vi "模态分析使用版.vi"() -> ()   [LabVIEW 2014]
uses:
  <vilib>/Analysis/4window.llb/windowTd.ctl
  <vilib>/Analysis/3filter.llb/Filter Structure Type.ctl
  <vilib>/measure/macond.llb/IIR Filter for 1 Chan.vi
  <vilib>/Waveform/WDTOps.llb/WDT Number of Waveform Samples DBL.vi
  <vilib>/Waveform/WDTOps.llb/WDT Append Waveforms DBL.vi
  <vilib>/Waveform/WDTOps.llb/WDT Get Waveform Subset DBL.vi
  <vilib>/measure/maspectr.llb/Frequency Response Function (Mag-Phase) 1-1.vi
  <vilib>/measure/NI_MAPro.lvlib
  <vilib>/Analysis/NI_AALPro.lvlib
  <vilib>/Analysis/NI_AALBase.lvlib
panel:
  out "数组 4":dbl[](array[numeric])
  out "数组 3":dbl[](array[numeric])
  out "FRF magnifitude 10":dbl[](graph) caption="FRF magnifitude"
  out "FRF magnifitude 8":cluster{"f0":dbl, "df":dbl, "magnitude":dbl[]}(graph) caption="FRF magnifitude"
  out "FRF magnifitude 7":cluster{"f0":dbl, "df":dbl, "magnitude":dbl[]}(graph) caption="FRF magnifitude"
  in  "filter structure option":T1=10 caption="滤波器结构选项" items=["IIR二阶"=0, "IIR四阶"=1, "自动选择"=10]
  in  "IIR filter specifications":T2={"Topology"=enum."Butterworth", "Type"=enum."Lowpass", "Order"=5, "Lower Fc"=1000.0, "Upper Fc"=200.0, "PB Ripple"=1.0, "SB Attenuation"=60.0} caption="IIR滤波器规范" {"PB Ripple" format="%0.2f"; "SB Attenuation" format="%0.2f"; "Lower Fc" format="%0.2p"; "Upper Fc" format="%0.2p"}
  out "FRF magnifitude 6":waveform(dbl)(graph) caption="FRF magnifitude"
  in  "Real":dbl
  out "FRF magnifitude 5":dbl[](graph) caption="FRF magnifitude"
  out "FRF magnifitude 3":cluster{"f0":dbl, "df":dbl, "magnitude":dbl[]}(graph) caption="FRF magnifitude"
  out "FRF magnifitude 2":cluster{"f0":dbl, "df":dbl, "magnitude":dbl[]}(graph) caption="FRF magnifitude"
  out "相关函数 2":cluster{"f0":dbl, "df":dbl, "magnitude":dbl[]}(graph)
  out "FRF Phase 2":cluster{"f0":dbl, "df":dbl, "magnitude":dbl[]}(graph)
  in  "FRF Mode 2":enum16{"H1", "H2", "H3"}(ring) caption="FRF模式"
  in  "averaging parameters 2":T3={"averaging mode"=enum."No averaging", "weighting mode"=enum."Exponential", "number of averages"=10} caption="平均参数" {"number of averages" min=1}
  out "error out 2":errorcluster caption="错误输出"
  in  "error in (no error)":errorcluster caption="错误输入（无错误）"
  in  "view 2":T4 caption="查看"
  in  "window 2":T5=1 caption="窗" items=["矩形"=0, "Hanning"=1, "Hamming"=2, "Blackman-Harris"=3, "Exact Blackman"=4, "Blackman"=5, "Flat Top"=6, "4阶Blackman-Harris "=7, "7阶Blackman-Harris"=8, "Low Sidelobe"=9, "Blackman Nuttall"=11, "三角"=30, "Bartlett-Hanning"=31, "Bohman"=32, "Parzen"=33, "Welch"=34, "Kaiser"=60, "Dolph-Chebyshev"=61, "高斯"=62]
  out "最大值":dbl
  out "数组 2":dbl[](array[numeric])
  out "数组":dbl[](array[numeric])
  out "error out":errorcluster
  in  "数值":i32
  out "FRF magnifitude":cluster{"f0":dbl, "df":dbl, "magnitude":dbl[]}(graph)
  out "相关函数":cluster{"f0":dbl, "df":dbl, "magnitude":dbl[]}(graph)
  out "FRF Phase":cluster{"f0":dbl, "df":dbl, "magnitude":dbl[]}(graph)
  out "响应信号":waveform(dbl)(graph)
  out "激振信号":waveform(dbl)(graph)
  in  "averaging parameters":T3={"averaging mode"=enum."No averaging", "weighting mode"=enum."Exponential", "number of averages"=10} caption="平均参数" {"number of averages" min=1}
  in  "window":T5=1 caption="窗" items=["矩形"=0, "Hanning"=1, "Hamming"=2, "Blackman-Harris"=3, "Exact Blackman"=4, "Blackman"=5, "Flat Top"=6, "4阶Blackman-Harris "=7, "7阶Blackman-Harris"=8, "Low Sidelobe"=9, "Blackman Nuttall"=11, "三角"=30, "Bartlett-Hanning"=31, "Bohman"=32, "Parzen"=33, "Welch"=34, "Kaiser"=60, "Dolph-Chebyshev"=61, "高斯"=62]
  in  "view":T4 caption="查看"
  in  "FRF Mode":enum16{"H1", "H2", "H3"}(ring) caption="FRF模式"
  in  "删除上一次波形":bool
  in  "激振计数":i32=-1 caption="预触发长度"
  in  "阈值":dbl=-1.0
  in  "预触发长度":i32=-1
  in  "激振通道":i32=-1
  in  "激振传感器灵敏度":dbl=-1.0
  in  "采集次数":i32=-1 caption="预触发长度"
  in  "停止按钮":bool
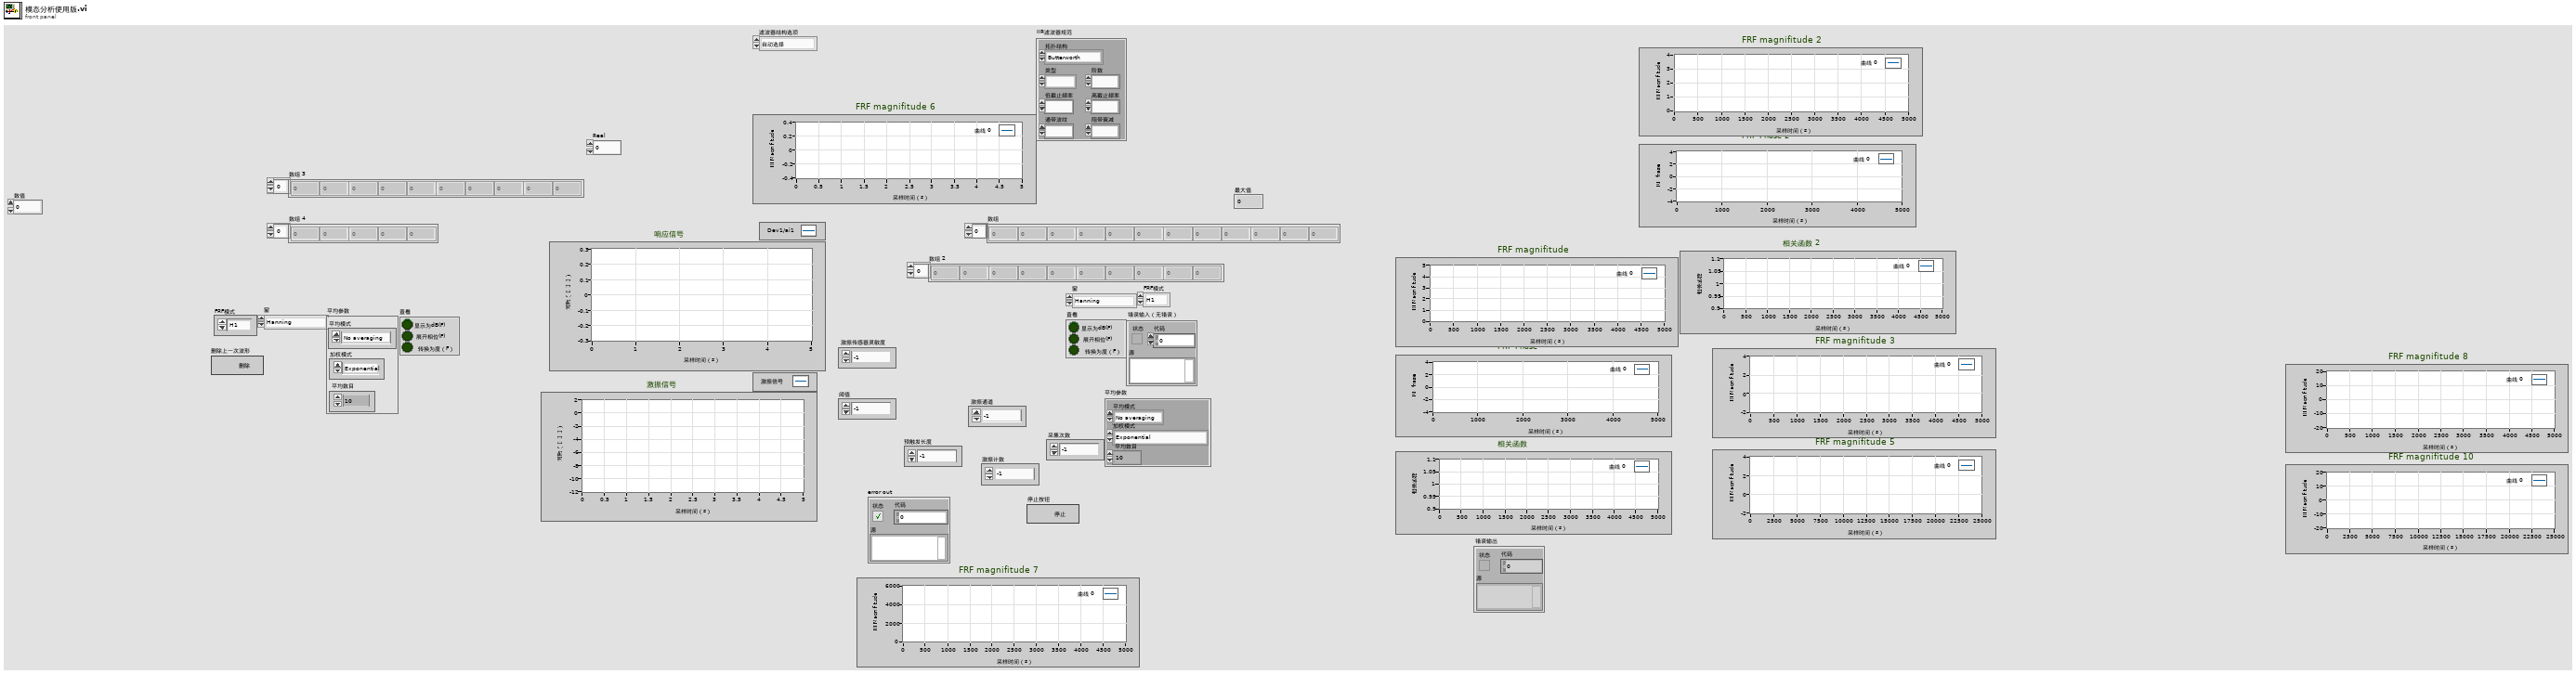
[diagram p1: front panel]
types:
  T1 = typedef "NI_AALBase.lvlib/Filter Structure Type.ctl" = u16
  T2 = cluster{"Topology":enum16{"Off", "Butterworth", "Chebyshev", "Inverse Chebyshev", "Elliptic", "Bessel"}, "Type":enum16{"Lowpass", "Highpass", "Bandpass", "Bandstop"}, "Order":i32, "Lower Fc":dbl, "Upper Fc":dbl, "PB Ripple":dbl, "SB Attenuation":dbl}
  T3 = cluster{"averaging mode":enum16{"No averaging", "Vector averaging", "RMS averaging", "Peak hold"}, "weighting mode":enum16{"Linear", "Exponential"}, "number of averages":u32}
  T4 = cluster{"dB On (F)":bool, "unwrap phase (F)":bool, "convert to degree (F)":bool}
  T5 = typedef "NI_AALPro.lvlib/windowTd.ctl" = u32
  T6 = cluster{"magnitude":cluster{"f0":dbl, "df":dbl, "magnitude":dbl[]}, "phase":cluster{"f0":dbl, "df":dbl, "phase":dbl[]}, "coherence":cluster{"f0":dbl, "df":dbl, "coherence":dbl[]}}
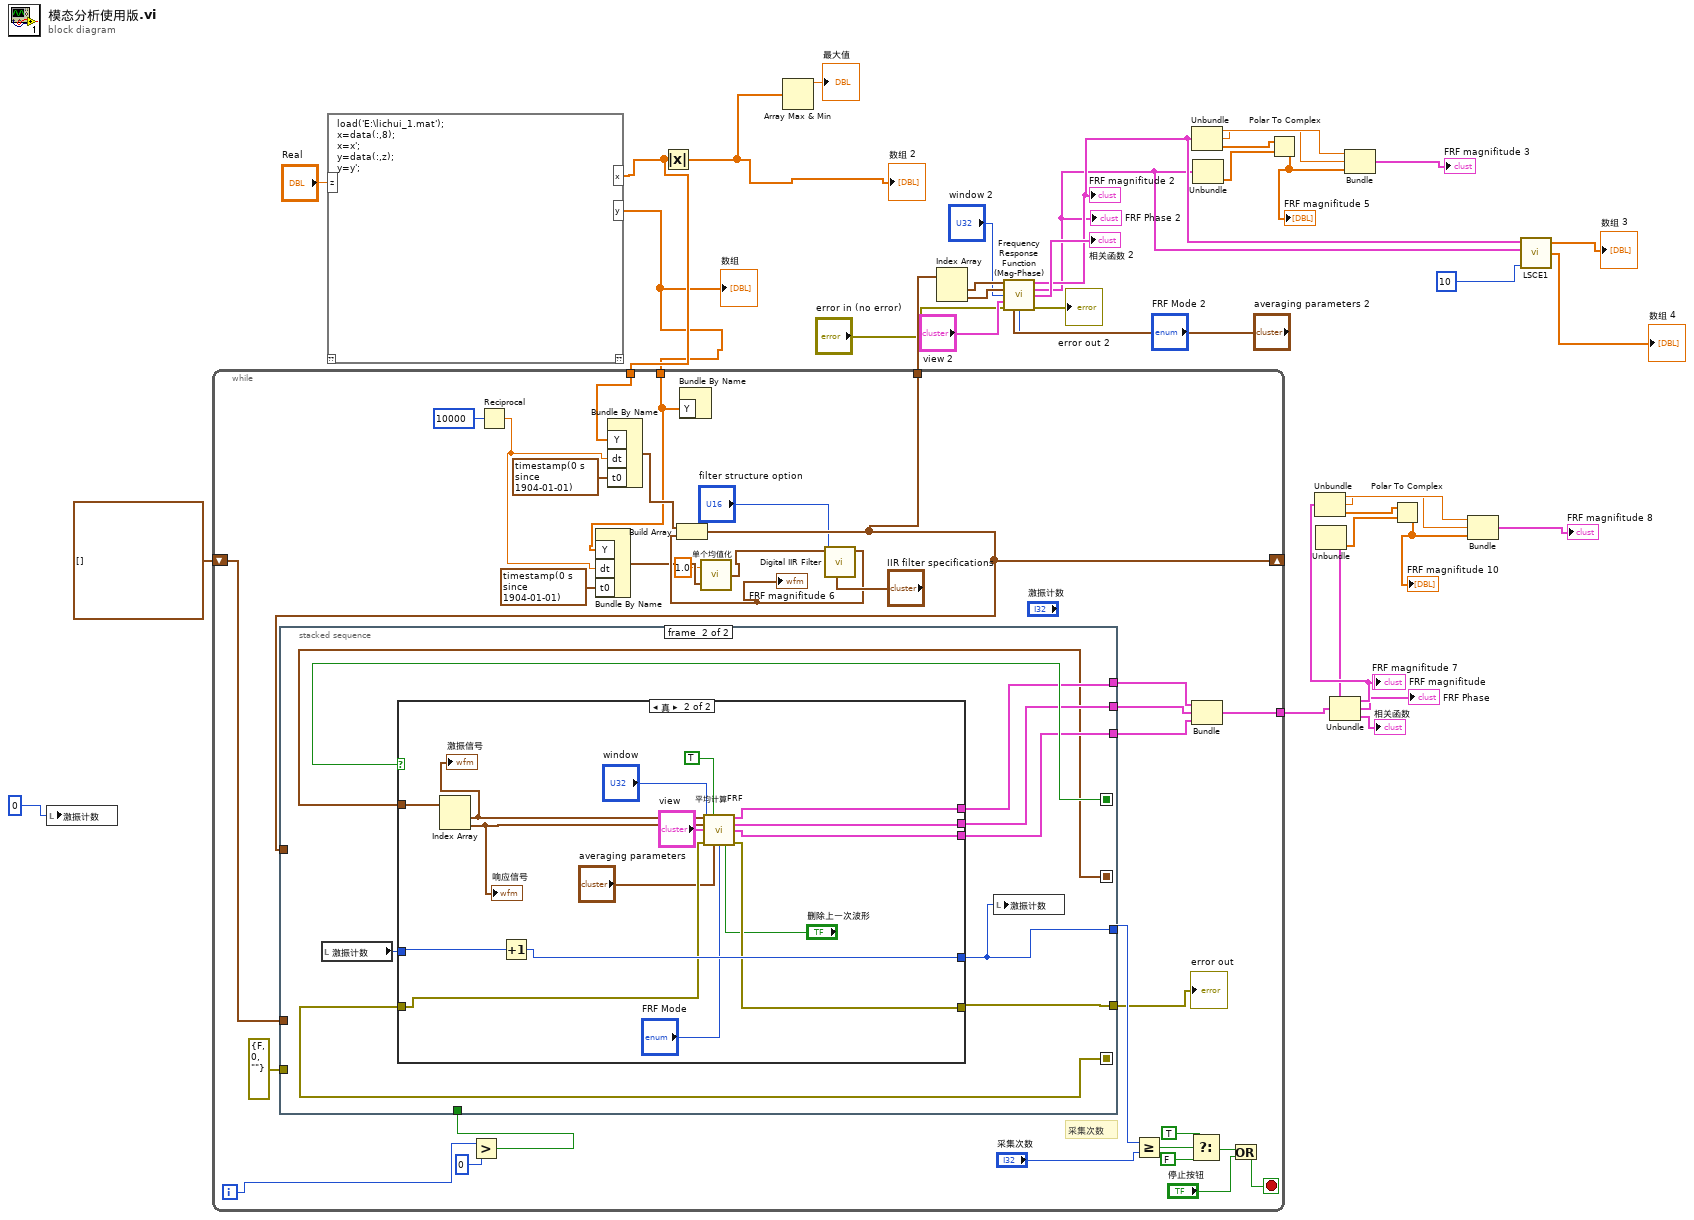
[diagram p0: block diagram]
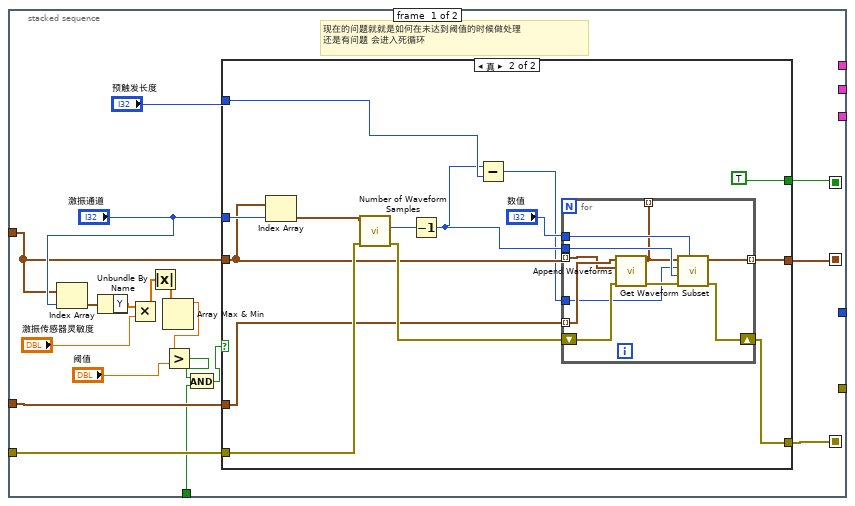
[diagram p2: hidden frame]
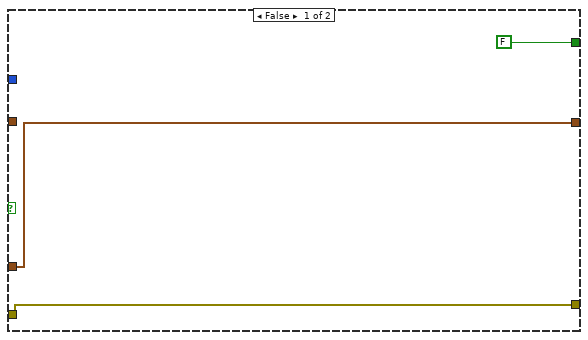
[diagram p3: hidden frame]
diagram:
  n1 = local write "激振计数"(0) -> ()
  n2 = script code="load('E:\\lichui_1.mat');\nx=data(:,8);\nx=x';\ny=data(:,z);\ny=y';"("z"="Real") -> ("x"=w15:dbl[], "y"=w14:dbl[])  [unwired: 1 in, 1 out]
  "数组" <- w14
  n3 = while {
    shift-right: [w47] -> _
    shift-left: waveform(dbl)[] [] ("data") -> [w70]
    tunnel: [w61] -> w35
    tunnel: w15 -> [w48]
    tunnel: w14 -> [w45]
    tunnel: [w47] -> w33
    i -> [w56]
    stop <- w59 stop-if-true
    # "采集次数"
    n4 = Greater?(x=w56, y=0) -> (0:w55:bool)
    n5 = Reciprocal(x=10000) -> (1/x=w49:dbl)
    n6 = Bundle By Name("Y"=w45, "dt"=w49, "t0"=timestamp(0 s since 1904-01-01)) -> (w41:waveform(dbl))  [unwired: 1 in]
    n7 = Bundle By Name("Y"=w48, "dt"=w49, "t0"=timestamp(0 s since 1904-01-01)) -> (w46:waveform(dbl))  [unwired: 1 in]
    n8 = Bundle By Name("Y"=w45) -> ()  [unwired: 1 in, 1 out]
    n9 = call "单个均值化.vi"("温度信号 4"=w41, "传感器灵敏度"=1.0) -> ("温度信号 3"=w40:waveform(dbl))
    n10 = call-poly <vilib>:"Digital IIR Filter.vi"("IIR filter specifications"="IIR filter specifications", "filter structure option"="filter structure option", "signal in"=w40) -> ("signal out"=w42:waveform(dbl))  [unwired: 6 in, 2 out]
    "FRF magnifitude 6" <- w42
    n11 = Build Array(w46, w42) -> (w47:waveform(dbl)[])
    n12 = stacked-sequence {
      seq-local: [w82 _] -> [_ w124]
      seq-local: [w81 _] -> [_ w117]
      seq-local: [w80 _] -> [_ w116]
      tunnel: w47 -> [w78 _]
      tunnel: w70 -> [w88 _]
      tunnel: errorcluster {"status"=FALSE, "code"=0, "source"=""} ("error out") -> [w79 _]
      tunnel: [_ w118] -> w66
      tunnel: [_ w122] -> w54
      tunnel: [_ w121] -> w64
      tunnel: [_ w120] -> w63
      tunnel: [_ w119] -> w62
      tunnel: w55 -> [w76 _]
      frame #0 {
        # "现在的问题就就是如何在未达到阈值的时候做处理\n还是有问题 会进入死循环"
        n13 = Index Array(array=w78, index="激振通道") -> (element=w86:waveform(dbl))
        n14 = Unbundle By Name(w86) -> ("Y"=w85:dbl[])
        n15 = Multiply(x=w85, y="激振传感器灵敏度") -> (x*y=w72:dbl[])
        n16 = Absolute Value(x=w72) -> (abs(x)=w71:dbl[])
        n17 = Array Max & Min(array=w71) -> (max value=w73:dbl)  [unwired: 3 out]
        n18 = Greater?(x=w73, y="阈值") -> (0:w75:bool)
        n19 = And(x=w75, y=w76) -> (x .and. y?=w74:bool)
        n20 = case shown="真" w74 {
          tunnel: w78 -> [_ w96]
          tunnel: "激振通道" -> [_ w105]
          tunnel: w79 -> [w91 w103]
          tunnel: "预触发长度" -> [_ w94]
          tunnel: w88 -> [w89 w95]
          tunnel: [w91 w101] -> w80
          tunnel: [w89 w99] -> w81
          tunnel: [FALSE TRUE] -> w82
          frame False {
          }
          frame True {
            n21 = Index Array(array=w96, index=w105) -> (element=w98:waveform(dbl))
            n22 = call-poly <vilib>:"Number of Waveform Samples.vi"("error in (no error)"=w103, "waveform in"=w98) -> ("error out"=w102:errorcluster, "number of samples"=w104:i32)  [unwired: 7 in, 1 out]
            n23 = Decrement(x=w104) -> (x-1=w93:i32)
            n24 = Subtract(x=w93, y=w94) -> (x-y=w92:i32)
            n25 = for {
              shift-right: [w110] -> w101
              shift-left: w102 -> [w113]
              tunnel: w96 -> [w114] mode=indexing
              tunnel: [w111] -> w99 mode=indexing
              tunnel: "数值" -> [w108]
              tunnel: w95 -> [w115] mode=indexing
              tunnel: w92 -> [w106]
              tunnel: w93 -> [w109]
              tunnel: [w107] -> _ mode=indexing
              n26 = call-poly <vilib>:"Append Waveforms.vi"("error in (no error)"=w113, "waveform B"=w114, "waveform A"=w115) -> ("error out"=w112:errorcluster, "waveform out"=w107:waveform(dbl))  [unwired: 7 in]
              n27 = call-poly <vilib>:"Get Waveform Subset.vi"("start/duration format"=w108, "error in (no error)"=w112, "duration"=w109, "start samples/time"=w106, "waveform in"=w107) -> ("error out"=w110:errorcluster, "waveform out"=w111:waveform(dbl))  [unwired: 1 in, 2 out]
            }
          }
        }
      }
      frame #1 {
        n28 = local read "激振计数"() -> (w123:i32)
        n29 = case shown="真" w124 {
          tunnel: w117 -> [_ w129]
          tunnel: w116 -> [w125 w140]
          tunnel: w123 -> [w126 w142]
          tunnel: [w126 w141] -> w118
          tunnel: [w125 w139] -> w122
          tunnel: [_ w132] -> w121
          tunnel: [_ w131] -> w120
          tunnel: [_ w130] -> w119
          frame False {
          }
          frame True {
            n30 = Index Array(array=w129) -> (element #1=w128:waveform(dbl), element #2=w127:waveform(dbl))  [unwired: 2 in]
            "激振信号" <- w128
            "响应信号" <- w127
            n31 = Increment(x=w142) -> (x+1=w141:i32)
            n32 = call "平均计算FRF.vi"("time signal X"=w128, "restart averaging (F)"=TRUE, "time signal Y"=w127, "window"="window", "view"="view", "error in (no error)"=w140, "averaging parameters"="averaging parameters", "FRF Mode"="FRF Mode", "删除上一波形"="删除上一次波形") -> ("magnitude"=w132:cluster{"f0":dbl, "df":dbl, "magnitude":dbl[]}, "phase"=w131:cluster{"f0":dbl, "df":dbl, "phase":dbl[]}, "coherence"=w130:cluster{"f0":dbl, "df":dbl, "coherence":dbl[]}, "error out"=w139:errorcluster)  [unwired: 1 in, 2 out]
          }
        }
        n33 = local write "激振计数"(w118) -> ()
      }
    }
    "error out" <- w54
    n34 = Greater Or Equal?(x=w66, y="采集次数") -> (x >= y?=w69:bool)
    n35 = Select(t=TRUE, s=w69, f=FALSE) -> (s? t:f=w60:bool)
    n36 = Bundle("magnitude"=w64, "phase"=w63, "coherence"=w62) -> (w61:T6)  [unwired: 1 in]
    n37 = Or(x=w60, y="停止按钮") -> (x .or. y?=w59:bool)
  }
  n38 = Absolute Value(x=w15) -> (abs(x)=w17:dbl[])
  "数组 2" <- w17
  n39 = Array Max & Min(array=w17) -> (max value=→"最大值":dbl)  [unwired: 3 out]
  n40 = Index Array(array=w33) -> (element #1=w32:waveform(dbl), element #2=w31:waveform(dbl))  [unwired: 2 in]
  n41 = call-poly <vilib>:"Frequency Response Function (Mag-Phase).vi"("time signal X"=w32, "time signal Y"=w31, "window"="window 2", "view"="view 2", "error in (no error)"="error in (no error)", "averaging parameters"="averaging parameters 2", "FRF Mode"="FRF Mode 2") -> ("magnitude"=w3:cluster{"f0":dbl, "df":dbl, "magnitude":dbl[]}, "phase"=w2:cluster{"f0":dbl, "df":dbl, "phase":dbl[]}, "coherence"=→"相关函数 2":cluster{"f0":dbl, "df":dbl, "coherence":dbl[]}, "error out"=→"error out 2":errorcluster)  [unwired: 3 in, 2 out]
  "FRF Phase 2" <- w2
  "FRF magnifitude 2" <- w3
  n42 = Unbundle(w3) -> ("f0"=w21:dbl, "df"=w20:dbl, "magnitude"=w23:dbl[])
  n43 = Unbundle(w2) -> ("phase"=w22:dbl[])  [unwired: 2 out]
  n44 = Polar To Complex(1:w22, 2:w23) -> (0:w18:cdb[])
  "FRF magnifitude 5" <- w18
  n45 = Unbundle(w35) -> ("magnitude"=w7:cluster{"f0":dbl, "df":dbl, "magnitude":dbl[]}, "phase"=w6:cluster{"f0":dbl, "df":dbl, "phase":dbl[]}, "coherence"=→"相关函数":cluster{"f0":dbl, "df":dbl, "coherence":dbl[]})
  "FRF Phase" <- w6
  "FRF magnifitude" <- w7
  n46 = Unbundle(w7) -> ("f0"=w11:dbl, "df"=w10:dbl, "magnitude"=w13:dbl[])
  n47 = Unbundle(w6) -> ("phase"=w12:dbl[])  [unwired: 2 out]
  n48 = Bundle("f0"=w21, "df"=w20, w18) -> (→"FRF magnifitude 3":cluster{"f0":dbl, "df":dbl, cdb[]})  [unwired: 1 in]
  n49 = Polar To Complex(1:w12, 2:w13) -> (0:w8:cdb[])
  "FRF magnifitude 10" <- w8
  n50 = Bundle("f0"=w11, "df"=w10, w8) -> (→"FRF magnifitude 8":cluster{"f0":dbl, "df":dbl, cdb[]})  [unwired: 1 in]
  n51 = call "LSCE1.vi"("数值输入控件"=10, "FRF Phase"=w2, "FRF magnifitude"=w3) -> ("模态阻尼比"=→"数组 4":dbl[], "模态频率"=→"数组 3":dbl[])  [unwired: 2 in]
